vi "Create New Handler.File.Text.vi"(6 "File Path":path, 7 "Handler.File.Text in":refnum<class "Handler.File.Text.lvclass">, 8 "error in (no error)":errorcluster, 10 "Name":string, 11 "Level":T1(ring)) -> (0 "error out":errorcluster, 3 "Handler.File.Text out":refnum<class "Handler.File.Text.lvclass">)   [LabVIEW 2017, in "Error Log.lvlib" / "Handler.File.Text.lvclass"]
uses:
  Handler.File.Text.lvclass
  \\192.168.1.40\Neosoft/Partage/Dossiers Personnels/BRO/DevTools_BR/wc/ErrorLog/src/Handler.File/Handler.File.lvclass
  Handler.File/Handler.File.lvclass
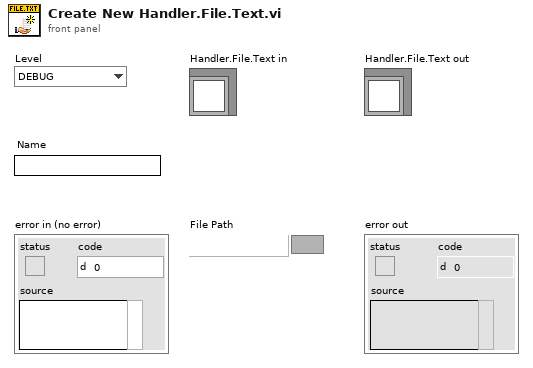
[diagram p1: front panel]
types:
  T1 = enum16{"DEBUG", "INFO", "WARNING", "ERROR", "CRITICAL"}
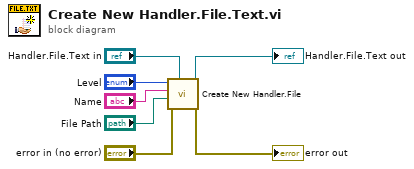
[diagram p0: block diagram]
diagram:
  n1 = call "Create New Handler.File.vi"("Handler.File in"="Handler.File.Text in", "error in (no error)"="error in (no error)", "File Path"="File Path", "Name"="Name", "Level"="Level") -> ("error out"=→"error out":errorcluster, "Handler.File out"=→"Handler.File.Text out":refnum<class "Handler.File.Text.lvclass">)  [unwired: 5 in]
